vi "Handle Dirty Flags.vi"(9 "Field IDs":T1[](array[typedef])) -> (2 "String out":string)   [LabVIEW 2017]
uses:
  <vilib>/Rock Robotics/Network Tables/Field ID.ctl
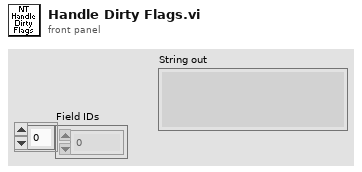
[diagram p1: front panel]
types:
  T1 = typedef "Field ID.ctl" = i32
  T2 = typedef "Field Data.ctl" = cluster{"Dbl":dbl, "String":string, "Type":T3, "Boolean":bool, "Sequence #":T4, "Flags":u8}
  T3 = typedef "Field Type.ctl" = enum8{"Invalid", "Bool", "Numeric", "String", "Raw", "Boolean Array", "Numeric Array", "String Array", "RPC"}
  T4 = typedef "Sequence.ctl" = u16
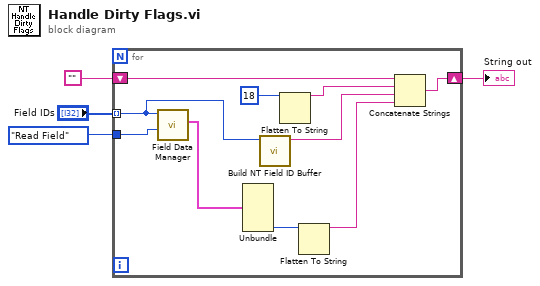
[diagram p0: block diagram]
diagram:
  n1 = for {
    tunnel: enum16{"Update Field", "Read Field"}."Read Field" ("Operation") -> [w14]
    tunnel: "Field IDs" -> [w10] mode=indexing
    shift-right: [w13] -> w4
    shift-left: "" -> [w12]
    n2 = call <vilib>:"Field Data Manager.vi"("Operation"=w14, "Field ID"=w10) -> ("Field Value Out"=w7:T2)  [unwired: 8 in, 1 out]
    n3 = Unbundle(w7) -> ("Flags"=w6:u8)  [unwired: 5 out]
    n4 = call <vilib>:"Build NT Field ID Buffer.vi"("Field ID"=w10) -> ("Data Buffer"=w8:string)  [unwired: 10 in]
    n5 = Flatten To String(anything=u8 18 ("bytes to read")) -> (data string=w9:string)  [unwired: 3 in, 2 out]
    n6 = Flatten To String(anything=w6) -> (data string=w5:string)  [unwired: 3 in, 2 out]
    n7 = Concatenate Strings(w12, w9, w8, w5) -> (w13:string)
  }
  "String out" <- w4
